vi "Animal_Deterrent_System.vi"() -> ()   [LabVIEW 2020]
uses:
  <vilib>/sound2/lvsound2.llb/Sound Output Task ID.ctl
  <vilib>/DAQmx/write.llb/DAQmx Write (Analog DBL 1Chan 1Samp).vi
  <vilib>/DAQmx/create/channels.llb/DAQmx Create Channel (AO-Voltage-Basic).vi
  <vilib>/DAQmx/miscellaneous.llb/DAQmx Fill In Error Info.vi
panel:
  out "output variable 2":dbl
  out "output variable 3":dbl
  in  "Boolean 2":bool
  in  "Boolean":bool
  out "element":path
  out "task ID":T1 format="%.0x"
  out "Avg":dbl
  in  "stop":bool
  out ".not. x?":bool
  out ".not. x? 2":bool
  out ".not. x? 4":bool
  out ".not. x? 3":bool
  out ".not. x? 6":bool
  out ".not. x? 5":bool
  out "x .and. y?":bool
  out "Light Output":dbl
  in  "physical channels 3":tag
  out "Piezo V":dbl format="%0.2f"
  out "Output variable":dbl
  out "PIR":dynamicdata(graph)
  out "Varying Peak":dbl
  out "Holding Peak":dbl
  out "IR_A":dbl
  out "IR_B":dbl
  in  "IR_A 4":bool
  in  "IR_B 5":bool
  out "Elephant 2":i32
  out "PeaFowl 2":u32
  out "Pig  2":u32
  out "Numeric 3":dbl
  in  "stop 2":bool
  out "True":bool
  out "False3":bool
  out "Pig1":bool
  out "Pig 2":bool
  out "Fowl 1":bool
  out "Fowl 2":bool
  out "Elephant 1":bool
  out "Eleplant 2":bool
  in  "Boolean 10":bool
  in  "Boolean 9":bool
  in  "Boolean 8":bool
  in  "Numeric 2":dbl
  in  "Boolean 7":bool
  out "Boolean 6":bool=TRUE
  in  "stop 3":bool
  # "ANIMAL DETERRENT SYSTEM"
  # "COUNT OF ANIMALS"
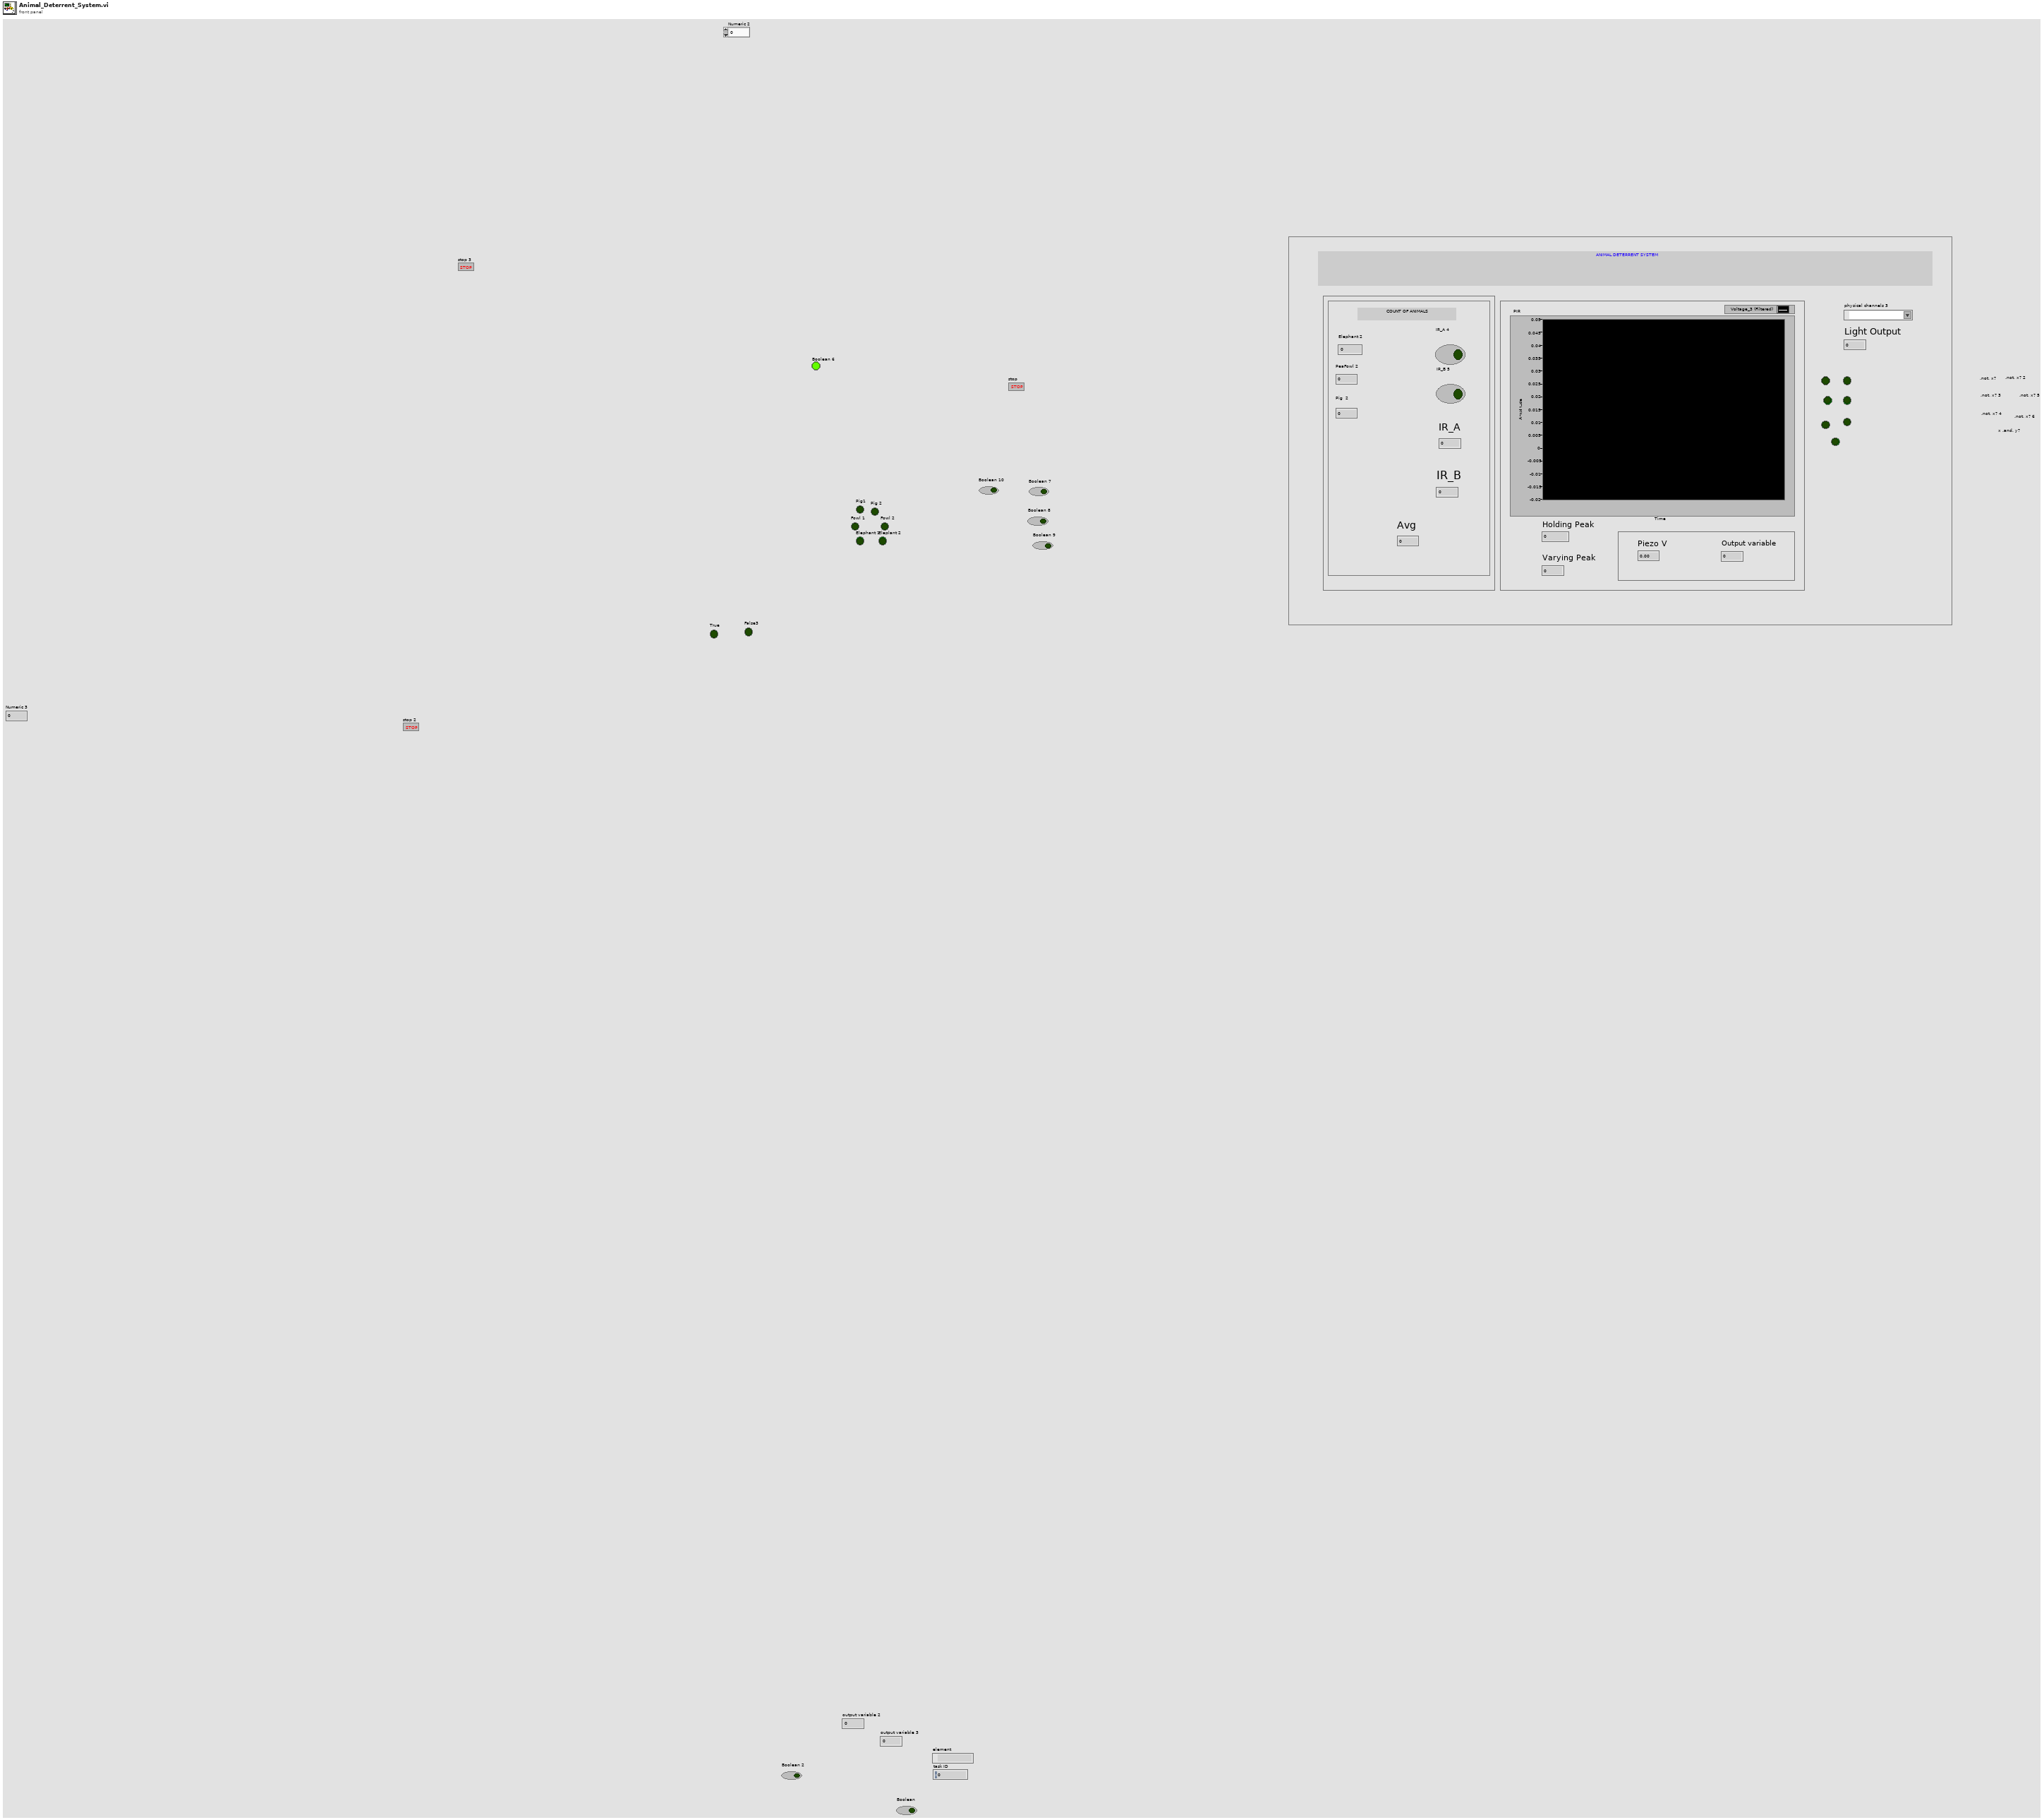
[diagram p1: front panel]
types:
  T1 = typedef "Sound Output Task ID.ctl" = u32
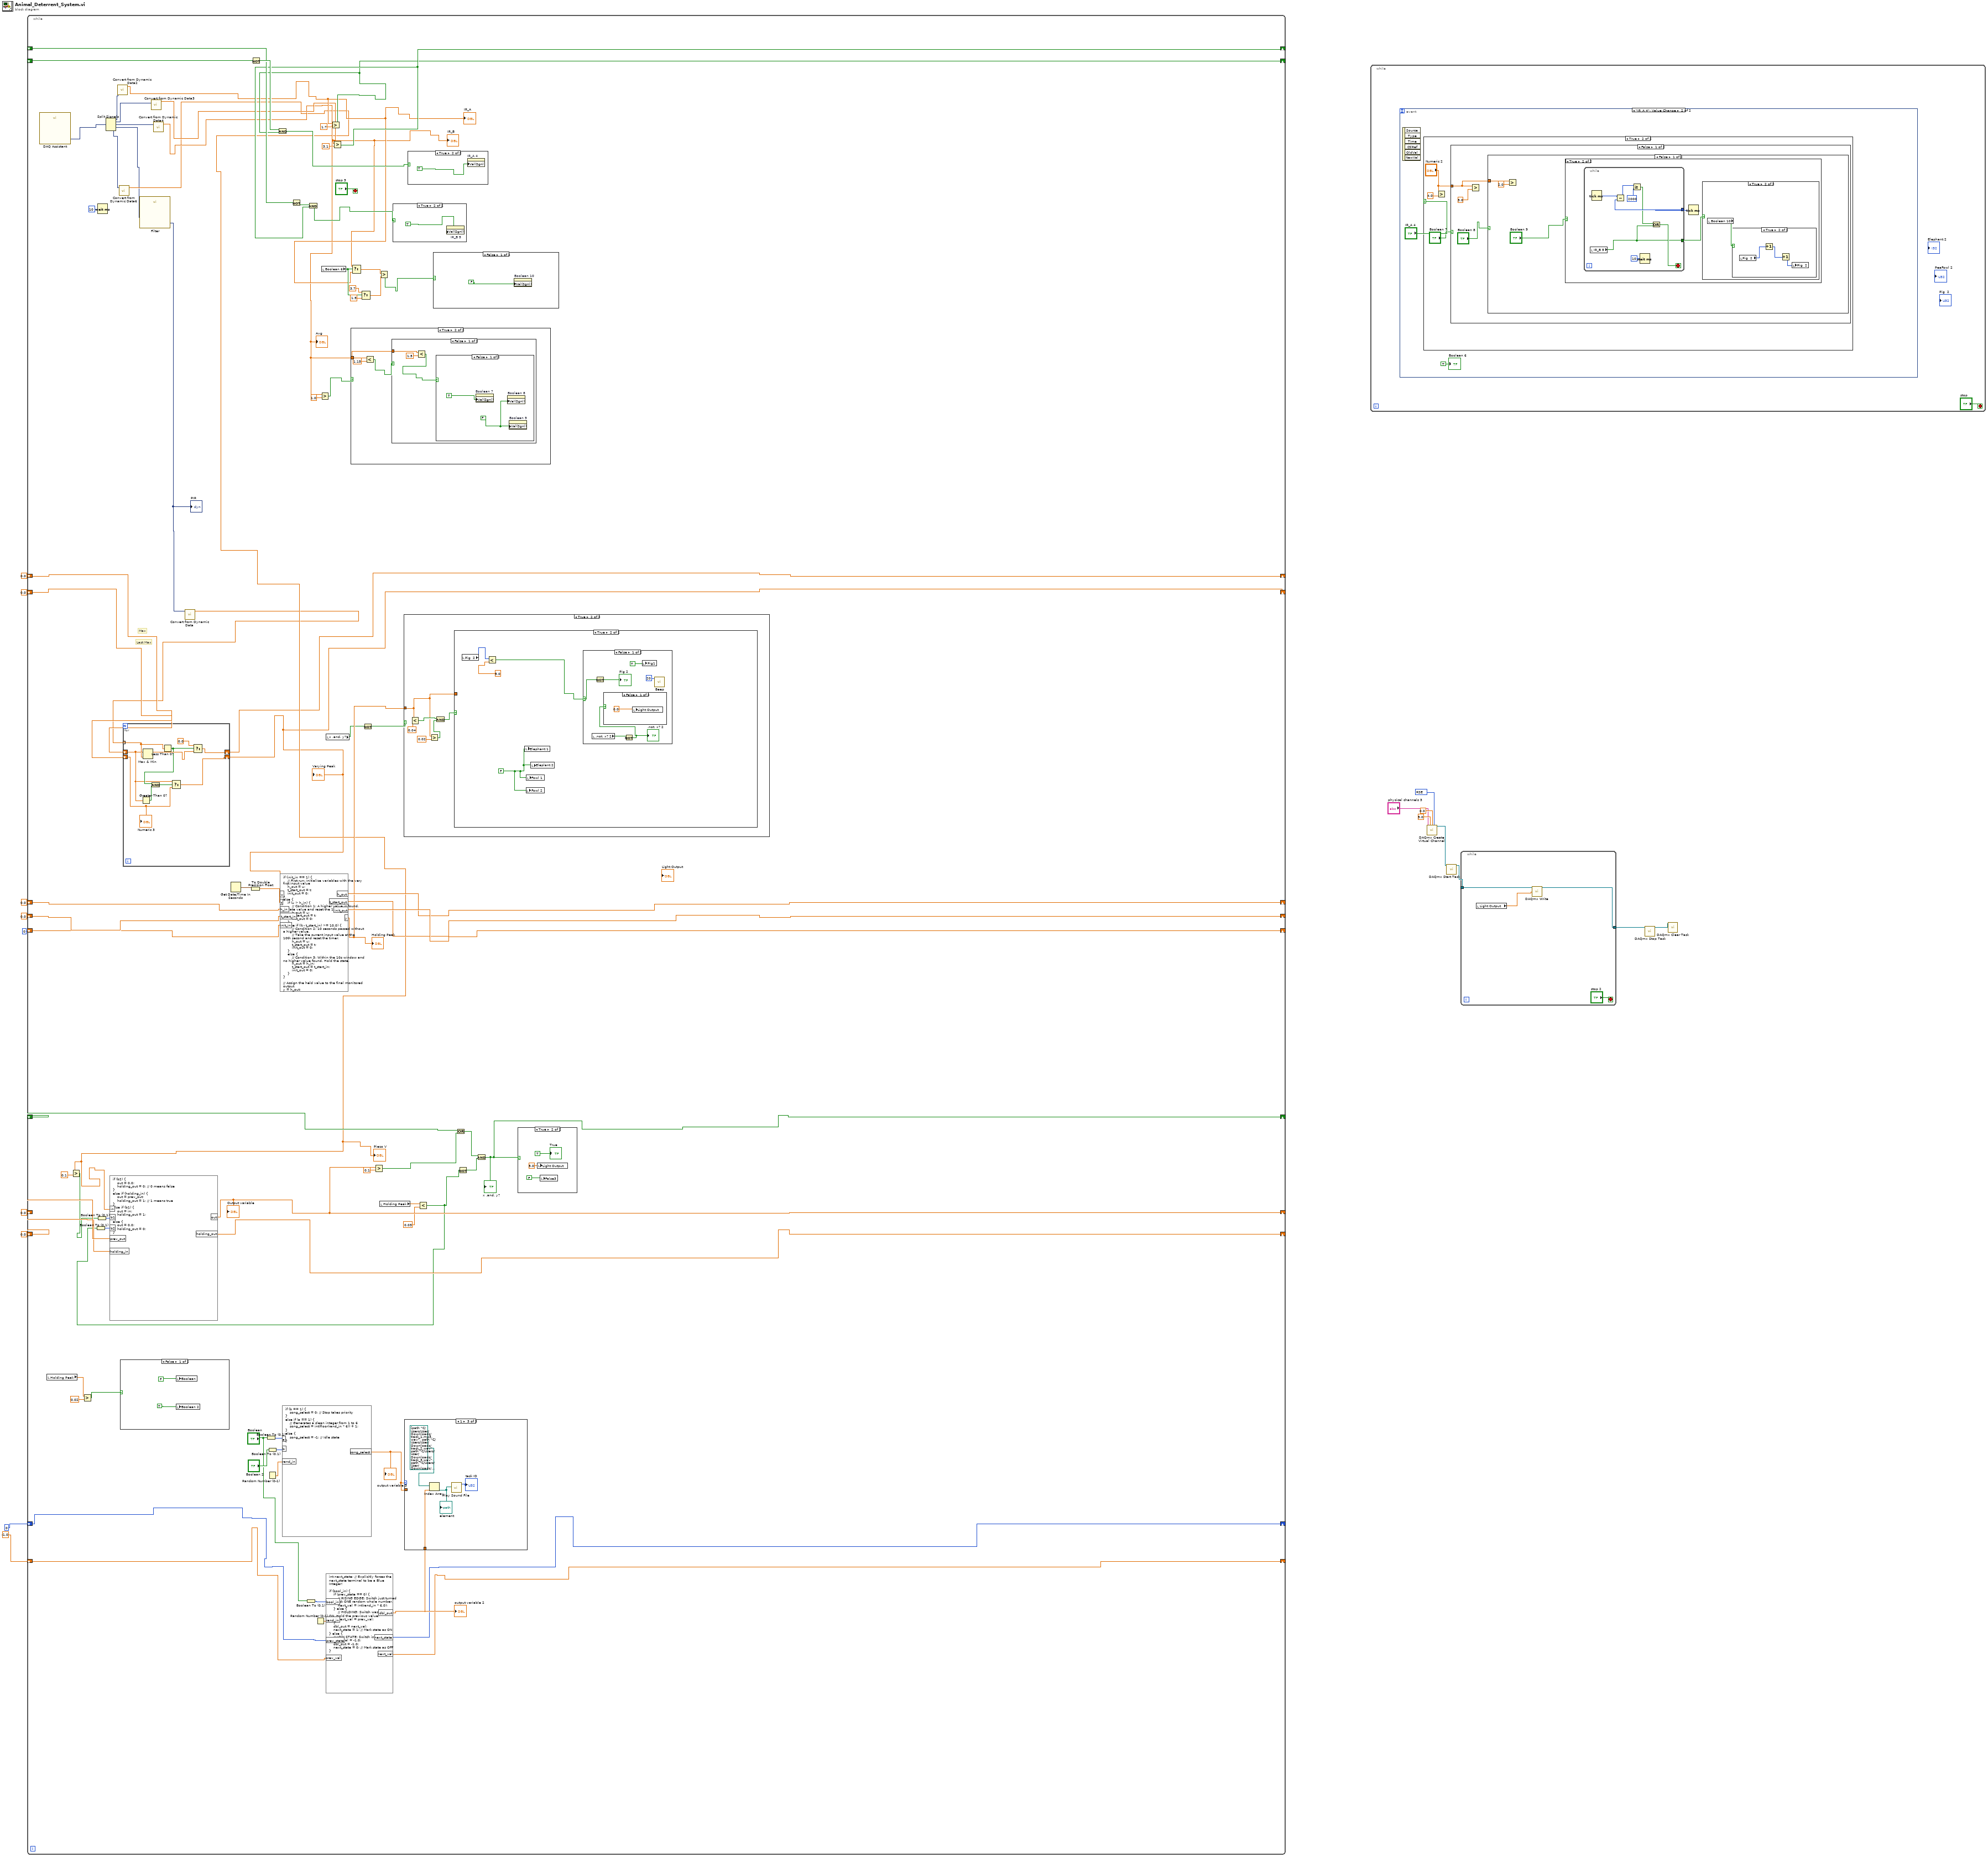
[diagram p0: block diagram]
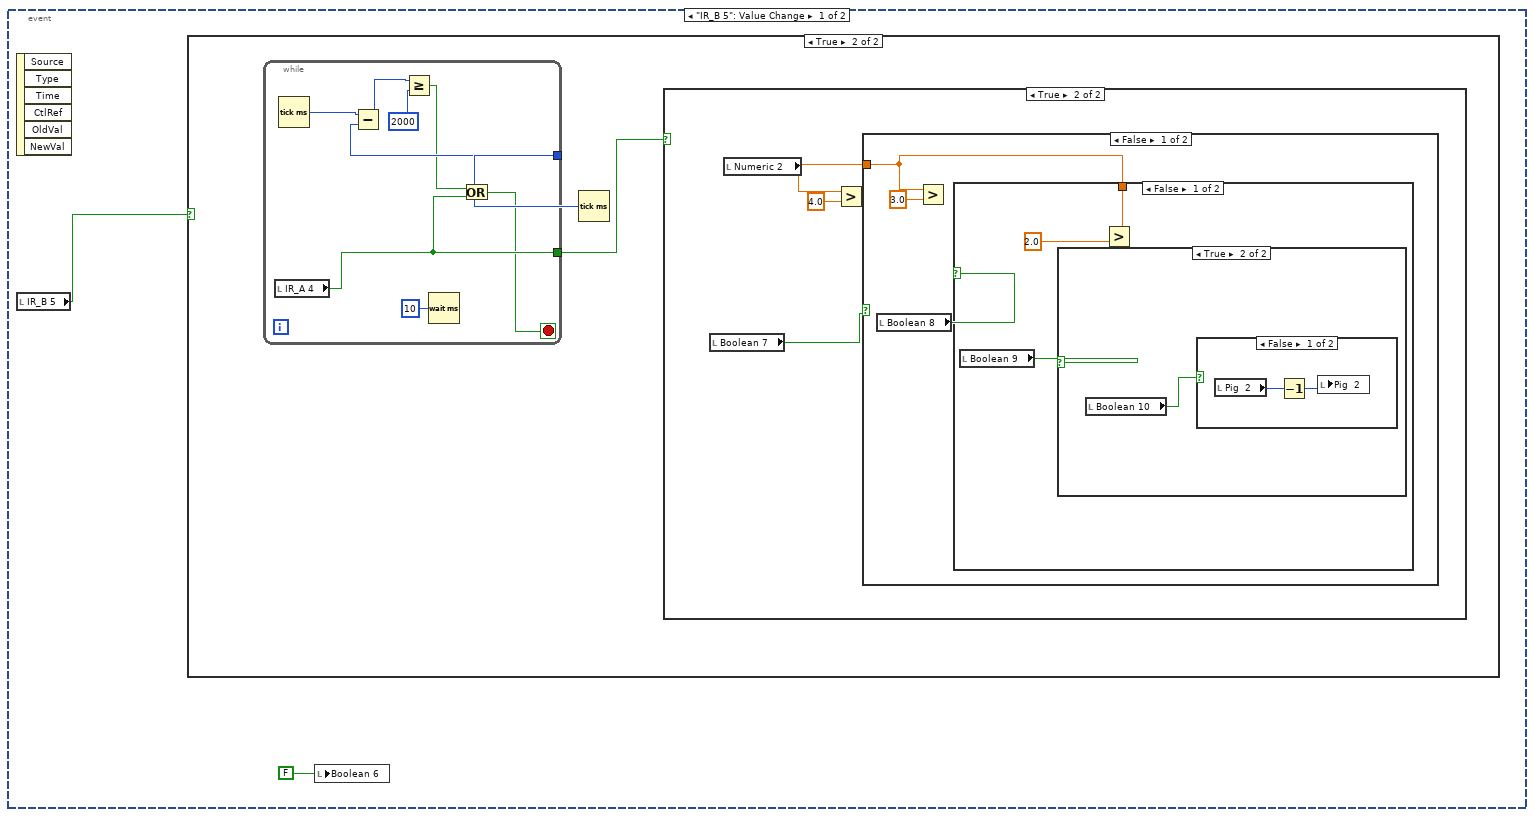
[diagram p2: hidden frame]
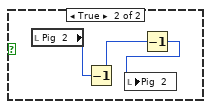
[diagram p6: hidden frame]
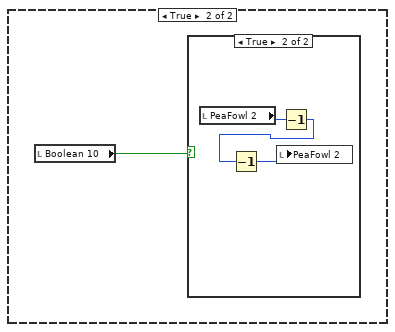
[diagram p7: hidden frame]
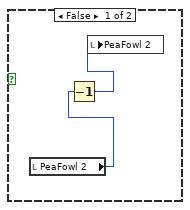
[diagram p8: hidden frame]
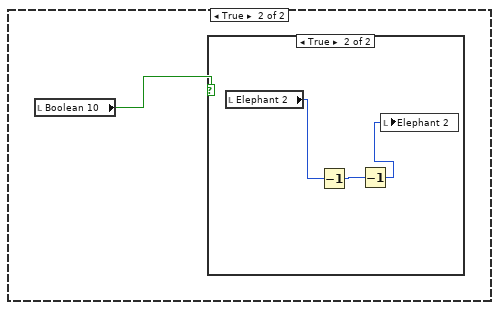
[diagram p9: hidden frame]
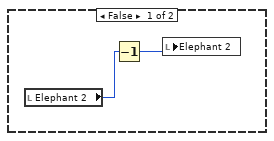
[diagram p10: hidden frame]
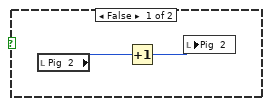
[diagram p14: hidden frame]
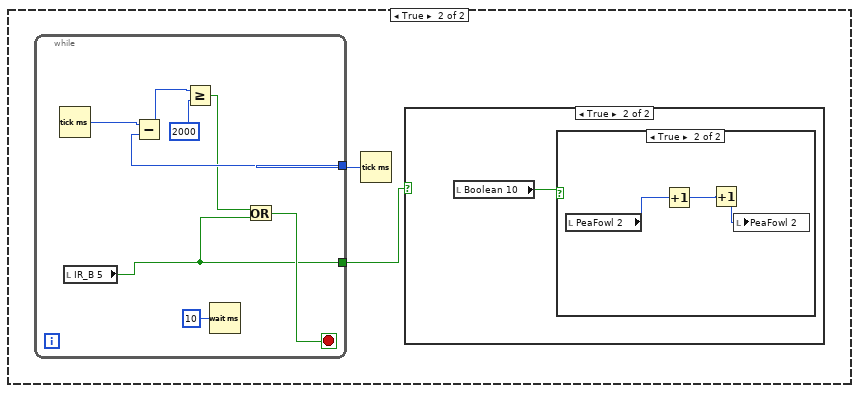
[diagram p15: hidden frame]
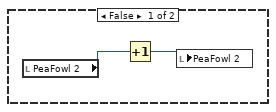
[diagram p17: hidden frame]
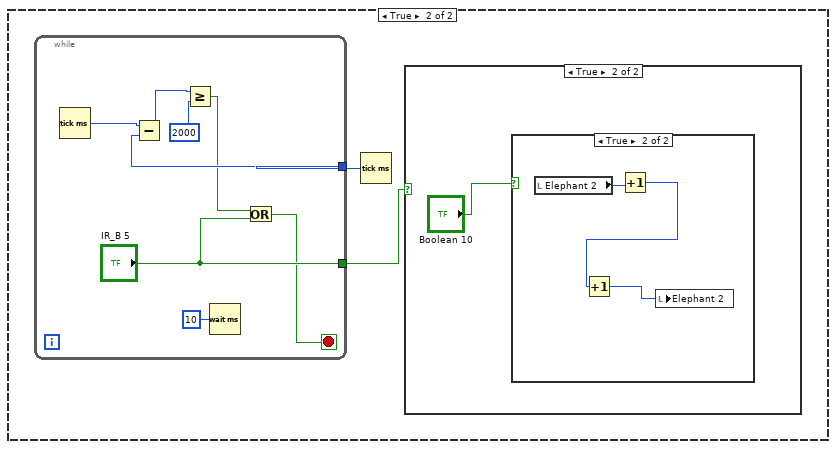
[diagram p18: hidden frame]
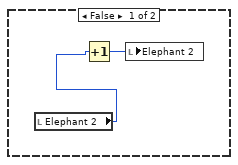
[diagram p20: hidden frame]
diagram:
  w6 = 10083 items=["Default"=-1, "RSE"=10083, "Differential"=10106, "Pseudodifferential"=12529] ("output terminal configuration")
  n1 = while {
    shift-right: [w55] -> _
    shift-left: _ -> [w94]
    shift-right: [w89] -> _
    shift-left: _ -> [w91]
    shift-right: [w41] -> _
    shift-left: 0.0 ("t") -> [w38]
    shift-right: [w40] -> _
    shift-left: 0.0 ("t") -> [w39]
    shift-right: [w71] -> _
    shift-left: 0.0 ("h_out") -> [w82]
    shift-right: [w72] -> _
    shift-left: 0.0 ("t_start_out") -> [w81]
    shift-right: [w73] -> _
    shift-left: 0 -> [w80]
    shift-right: [w74] -> _
    shift-left: _ -> [w79]
    shift-right: [w75] -> _
    shift-left: 0.0 ("out") -> [w78]
    shift-right: [w76] -> _
    shift-left: 0.0 ("holding_out") -> [w77]
    shift-right: [w22] -> _
    shift-left: 0 -> [w24]
    shift-right: [w21] -> _
    shift-left: -1.0 -> [w23]
    stop <- "stop 3" stop-if-true
    # "Last Max"
    # "Max"
    n2 = call "DAQ Assistant"() -> ("data"=w34:dynamicdata)  [unwired: 16 in, 3 out]
    n3 = local read "Holding Peak"() -> (w19:dbl)
    n4 = Greater?(x=w19, y=0.02) -> (0:w18:bool)
    n5 = Wait (ms)(milliseconds to wait=u32 10) -> ()  [unwired: 1 out]
    n6 = Split Signals(w34) -> (w47:dynamicdata, w50:dynamicdata, w49:dynamicdata, w42:dynamicdata, w48:dynamicdata)  [unwired: 5 in]
    n7 = call "Convert from Dynamic Data2"("Dynamic Data Type"=w47) -> ("Scalar"=w46:dbl)  [unwired: 3 in]
    "IR_A" <- w46
    n8 = call "Convert from Dynamic Data6"("Dynamic Data Type"=w48) -> ("Scalar"=w43:dbl)  [unwired: 3 in]
    "Piezo V" <- w43
    n9 = Greater?(x=w43, y=0.1) -> (0:w51:bool)
    n10 = Boolean To (0,1)(Boolean=w51) -> (0, 1=w62:i16)
    n11 = case shown="False" w18 {
      frame False {
        n12 = local write "Boolean"(FALSE) -> ()
        n13 = local write "Boolean 2"(TRUE) -> ()
      }
      frame True {
        n14 = local write "Boolean"(TRUE) -> ()
        n15 = local write "Boolean 2"(FALSE) -> ()
      }
    }
    n16 = call "Filter"("Signal"=w42) -> ("Filtered Signal"=w35:dynamicdata)  [unwired: 9 in, 1 out]
    "PIR" <- w35
    n17 = call "Convert from Dynamic Data3"("Dynamic Data Type"=w50) -> ("Scalar"=w45:dbl)  [unwired: 3 in]
    "IR_B" <- w45
    n18 = call "Convert from Dynamic Data4"("Dynamic Data Type"=w49) -> ("Scalar"=w44:dbl)  [unwired: 3 in]
    "Avg" <- w44
    n19 = call "Convert from Dynamic Data"("Dynamic Data Type"=w35) -> ("Array"=w36:dbl[])  [unwired: 3 in]
    n20 = for {
      shift-right: [w113] -> w41
      shift-left: w38 -> [w109]
      shift-right: [w107] -> w40
      shift-left: w39 -> [w108]
      tunnel: w36 -> [w115] mode=indexing
      n21 = Greater Than 0?(x=w109) -> (x > 0?=w112:bool)
      n22 = Max & Min(x=w115, y=w109) -> (max(x,y)=w116:dbl)  [unwired: 1 out]
      n23 = Less Than 0?(x=w115) -> (x < 0?=w111:bool)
      n24 = And(x=w111, y=w112) -> (x .and. y?=w110:bool)
      n25 = Select(t=w109, s=w110, f=w108) -> (s? t:f=w107:dbl)
      n26 = Select(t=0.0, s=w111, f=w116) -> (s? t:f=w113:dbl)
      "Numeric 3" <- w108
    }
    "Varying Peak" <- w40
    n27 = Get Date/Time In Seconds() -> (seconds since 1Jan1904=w70:timestamp)
    n28 = To Double Precision Float(number=w70) -> (double precision float=w69:dbl)
    n29 = Not(x=w94) -> (.not. x?=w93:bool)
    n30 = Boolean To (0,1)(Boolean="Boolean") -> (0, 1=w32:i16)
    n31 = Boolean To (0,1)(Boolean="Boolean 2") -> (0, 1=w31:i16)
    n32 = Random Number (0-1)() -> (number: 0 to 1=w29:dbl)
    n33 = formula code="if (init_in == 1) {\n    // First run: Initialize variables with the very first input value\n    h_out = u;\n    t_start_out = t;\n    init_out = 0;\n} \nelse {\n    if (u > h_in) {\n        // Condition 1: A higher value is found. Update value and reset the 10s timer.\n        h_out = u;\n        t_start_out = t;\n        init_out = 0;\n    } \n    else if ((t - t_start_in) >= 10.0) {\n        // Condition 2: 10 seconds passed without a higher value. \n        // Take the current input value at the 10th second and reset the timer.\n        h_out = u;\n        t_start_out = t;\n        init_out = 0;\n    } \n    else {\n        // Condition 3: Within the 10s window and no higher value found. Hold the state.\n        h_out = h_in;\n        t_start_out = t_start_in;\n        init_out = 0;\n    }\n}\n\n// Assign the held value to the final monitored output\ny = h_out;"("u"=w40, "t"=w69, "h_in"=w82, "t_start_in"=w81, "init_in"=w80) -> ("h_out"=w71:dbl, "t_start_out"=w72:dbl, "init_out"=w73:dbl, "y"=w68:dbl)
    "Holding Peak" <- w68
    n34 = formula code="if (b == 1) {\n    song_select = 0; // Stop takes priority\n} \nelse if (a == 1) {\n    // Generates a clean integer from 1 to 6\n    song_select = int(floor(rand_in * 6)) + 1; \n} \nelse {\n    song_select = -1; // Idle state\n}"("a"=w32, "b"=w31, "rand_in"=w29) -> ("song_select"=w33:dbl)
    "output variable 3" <- w33
    n35 = Not(x=w91) -> (.not. x?=w90:bool)
    n36 = Boolean To (0,1)(Boolean="Boolean") -> (0, 1=w28:i16)
    n37 = Random Number (0-1)() -> (number: 0 to 1=w27:dbl)
    n38 = Greater?(x=w44, y=1.0) -> (0:w52:bool)
    n39 = local read "Boolean 6"() -> (w83:bool)
    n40 = local read "x .and. y?"() -> (w56:bool)
    n41 = formula code="int next_state; // Explicitly forces the next_state terminal to be a Blue Integer!\n\nif (bool_in) {\n    if (prev_state == 0) {\n        // RISING EDGE: Switch just turned ON. Pick ONE random whole number.\n        next_val = int(rand_in * 6.0);\n    } else {\n        // HOLDING: Switch was already ON. Hold the previous value.\n        next_val = prev_val;\n    }\n    dbl_out = next_val;\n    next_state = 1; // Mark state as ON\n} else {\n    // LOW STATE: Switch is OFF.\n    next_val = -1.0;\n    dbl_out = -1.0;\n    next_state = 0; // Mark state as OFF\n}"("bool_in"=w28, "rand_in"=w27, "prev_state"=w24, "prev_val"=w23) -> ("dbl_out"=w26:dbl, "next_state"=w22:i32, "next_val"=w21:dbl)
    "output variable 2" <- w26
    n42 = Greater?(x=w46, y=1.7) -> (0:w55:bool)
    n43 = And(x=w93, y=w55) -> (x .and. y?=w92:bool)
    n44 = Greater?(x=w45, y=3.1) -> (0:w89:bool)
    n45 = And(x=w90, y=w89) -> (x .and. y?=w54:bool)
    n46 = case shown="True" w52 {
      tunnel: w44 -> [_ w200]
      frame False {
      }
      frame True {
        n47 = Less?(x=w200, y=1.15) -> (x < y?=w199:bool)
        n48 = case shown="False" w199 {
          tunnel: w200 -> [w203 _]
          frame False {
            n49 = Less?(x=w203, y=1.5) -> (x < y?=w202:bool)
            n50 = case shown="False" w202 {
              frame False {
                w205 = FALSE
                n51 = property on="Boolean 7" class="Bool (strict)"("Val(Sgnl)"=TRUE) -> ()  [unwired: 2 in, 2 out]
                n52 = property on="Boolean 8" class="Bool (strict)"("Val(Sgnl)"=w205) -> ()  [unwired: 2 in, 2 out]
                n53 = property on="Boolean 9" class="Bool (strict)"("Val(Sgnl)"=w205) -> ()  [unwired: 2 in, 2 out]
              }
              frame True {
                w207 = FALSE
                n54 = property on="Boolean 8" class="Bool (strict)"("Val(Sgnl)"=TRUE ("Value (Signaling)")) -> ()  [unwired: 2 in, 2 out]
                n55 = property on="Boolean 9" class="Bool (strict)"("Val(Sgnl)"=w207) -> ()  [unwired: 2 in, 2 out]
                n56 = property on="Boolean 7" class="Bool (strict)"("Val(Sgnl)"=w207) -> ()  [unwired: 2 in, 2 out]
              }
            }
          }
          frame True {
            w209 = FALSE
            n57 = property on="Boolean 9" class="Bool (strict)"("Val(Sgnl)"=TRUE) -> ()  [unwired: 2 in, 2 out]
            n58 = property on="Boolean 7" class="Bool (strict)"("Val(Sgnl)"=w209) -> ()  [unwired: 2 in, 2 out]
            n59 = property on="Boolean 8" class="Bool (strict)"("Val(Sgnl)"=w209) -> ()  [unwired: 2 in, 2 out]
          }
        }
      }
    }
    n60 = Select(t=w45, s=w83, f=w46) -> (s? t:f=w87:dbl)
    n61 = Select(t=3.7 ("y"), s=w83, f=1.9) -> (s? t:f=w84:dbl)
    n62 = Not(x=w56) -> (.not. x?=w57:bool)
    n63 = Greater?(x=w87, y=w84) -> (0:w53:bool)
    n64 = local read "Holding Peak"() -> (w64:dbl)
    n65 = case shown="True" w54 {
      frame False {
        n66 = property on="IR_B 5" class="Bool (strict)"("Val(Sgnl)"=FALSE) -> ()  [unwired: 2 in, 2 out]
      }
      frame True {
        n67 = property on="IR_B 5" class="Bool (strict)"("Val(Sgnl)"=TRUE) -> ()  [unwired: 2 in, 2 out]
      }
    }
    n68 = case shown="True" w57 {
      tunnel: w68 -> [_ w117]
      frame False {
      }
      frame True {
        n69 = Less?(x=w117, y=0.04) -> (x < y?=w120:bool)
        n70 = Greater?(x=w117, y=0.02) -> (0:w119:bool)
        n71 = And(x=w120, y=w119) -> (x .and. y?=w118:bool)
        n72 = case shown="True" w118 {
          tunnel: w117 -> [w126 _]
          frame False {
            n73 = Less?(x=w126, y=0.1) -> (x < y?=w124:bool)
            n74 = Greater?(x=w126, y=0.04) -> (0:w127:bool)
            n75 = And(x=w127, y=w124) -> (x .and. y?=w123:bool)
            n76 = case shown="True" w123 {
              tunnel: w126 -> [w130 _]
              frame False {
                n77 = Greater?(x=w130, y=0.1) -> (0:w129:bool)
                n78 = case shown="True" w129 {
                  frame False {
                    n79 = local write "Light Output"(0.0) -> ()
                  }
                  frame True {
                    w134 = TRUE
                    w135 = TRUE
                    n80 = local read "Elephant 2"() -> (w133:i32)
                    n81 = local write "Fowl 1"(w134) -> ()
                    n82 = Less?(x=w133, y=5.0) -> (x < y?=w136:bool)
                    n83 = local write "Fowl 2"(w134) -> ()
                    n84 = case shown="True" w136 {
                      selector: w136 -> [w143 w150]
                      frame False {
                        n85 = local read ".not. x? 5"() -> (w140:bool)
                        n86 = Not(x=w140) -> (.not. x?=w139:bool)
                        ".not. x? 5" <- w139
                        n87 = call <vilib>:"Beep.vi"("frequency (Hz)"=u32 60) -> ()  [unwired: 11 in]
                        n88 = case shown="True" w139 {
                          frame False {
                            n89 = local write "Light Output"(0.0 ("Light Output")) -> ()
                          }
                          frame True {
                            n90 = local write "Light Output"(3.75) -> ()
                          }
                        }
                        n91 = Not(x=w143) -> (.not. x?=→"Eleplant 2":bool)
                        n92 = local write "Elephant 1"(TRUE) -> ()
                      }
                      frame True {
                        n93 = local read ".not. x? 6"() -> (w148:bool)
                        n94 = Not(x=w148) -> (.not. x?=w147:bool)
                        ".not. x? 6" <- w147
                        n95 = case shown="True" w147 {
                          frame False {
                            n96 = local write "Light Output"(0.0 ("Light Output")) -> ()
                          }
                          frame True {
                            n97 = local write "Light Output"(3.6) -> ()
                          }
                        }
                        n98 = call <vilib>:"Beep.vi"("frequency (Hz)"=u32 50) -> ()  [unwired: 11 in]
                        n99 = local write "Eleplant 2"(FALSE) -> ()
                        "Elephant 1" <- w150
                      }
                    }
                    n100 = local write "Pig 2"(w135) -> ()
                    n101 = local write "Pig1"(w135) -> ()
                  }
                }
              }
              frame True {
                w154 = FALSE
                w155 = TRUE
                n102 = local read "PeaFowl 2"() -> (w153:u32)
                n103 = local write "Eleplant 2"(w154) -> ()
                n104 = local write "Elephant 1"(w154) -> ()
                n105 = Less?(x=w153, y=5.0) -> (x < y?=w156:bool)
                n106 = case shown="True" w156 {
                  selector: w156 -> [w163 w170]
                  frame False {
                    n107 = call <vilib>:"Beep.vi"("frequency (Hz)"=u32 40) -> ()  [unwired: 11 in]
                    n108 = local read ".not. x? 3"() -> (w160:bool)
                    n109 = Not(x=w163) -> (.not. x?=→"Fowl 2":bool)
                    n110 = Not(x=w160) -> (.not. x?=w159:bool)
                    ".not. x? 3" <- w159
                    n111 = case shown="True" w159 {
                      frame False {
                        n112 = local write "Light Output"(0.0 ("Light Output")) -> ()
                      }
                      frame True {
                        n113 = local write "Light Output"(3.45 ("Light Output")) -> ()
                      }
                    }
                    n114 = local write "Fowl 1"(TRUE) -> ()
                  }
                  frame True {
                    n115 = local read ".not. x? 4"() -> (w168:bool)
                    n116 = call <vilib>:"Beep.vi"("frequency (Hz)"=u32 30) -> ()  [unwired: 11 in]
                    n117 = Not(x=w168) -> (.not. x?=w167:bool)
                    ".not. x? 4" <- w167
                    n118 = case shown="True" w167 {
                      frame False {
                        n119 = local write "Light Output"(0.0 ("Light Output")) -> ()
                      }
                      frame True {
                        n120 = local write "Light Output"(3.3 ("Light Output")) -> ()
                      }
                    }
                    n121 = local write "Fowl 2"(FALSE) -> ()
                    "Fowl 1" <- w170
                  }
                }
                n122 = local write "Pig 2"(w155) -> ()
                n123 = local write "Pig1"(w155) -> ()
              }
            }
          }
          frame True {
            w174 = FALSE
            n124 = local read "Pig  2"() -> (w173:u32)
            n125 = Less?(x=w173, y=5.0) -> (x < y?=w175:bool)
            n126 = local write "Elephant 1"(w174) -> ()
            n127 = local write "Fowl 2"(w174) -> ()
            n128 = local write "Fowl 1"(w174) -> ()
            n129 = local write "Eleplant 2"(w174) -> ()
            n130 = case shown="False" w175 {
              selector: w175 -> [w182 w189]
              frame False {
                n131 = local read ".not. x? 2"() -> (w180:bool)
                n132 = Not(x=w182) -> (.not. x?=→"Pig 2":bool)
                n133 = Not(x=w180) -> (.not. x?=w179:bool)
                ".not. x? 2" <- w179
                n134 = case shown="False" w179 {
                  frame False {
                    n135 = local write "Light Output"(0.0) -> ()
                  }
                  frame True {
                    n136 = local write "Light Output"(1.8) -> ()
                  }
                }
                n137 = local write "Pig1"(TRUE) -> ()
                n138 = call <vilib>:"Beep.vi"("frequency (Hz)"=u32 20) -> ()  [unwired: 11 in]
              }
              frame True {
                n139 = local read ".not. x?"() -> (w187:bool)
                n140 = Not(x=w187) -> (.not. x?=w186:bool)
                ".not. x?" <- w186
                n141 = case shown="True" w186 {
                  frame False {
                    n142 = local write "Light Output"(0.0 ("Light Output")) -> ()
                  }
                  frame True {
                    n143 = local write "Light Output"(1.6) -> ()
                  }
                }
                n144 = local write "Pig 2"(FALSE) -> ()
                n145 = call <vilib>:"Beep.vi"("frequency (Hz)"=u32 10) -> ()  [unwired: 11 in]
                "Pig1" <- w189
              }
            }
          }
        }
      }
    }
    n146 = case shown="1" w33 {
      tunnel: w33 -> [_ _ _]
      tunnel: w26 -> [_ _ w105]
      frame 0 {
        n147 = local read "task ID"() -> (w102:T1)
        n148 = call <vilib>:"Sound Output Stop.vi"("task ID"=w102) -> ()  [unwired: 9 in, 2 out]
      }
      frame Default {
      }
      frame 1 {
        n149 = Index Array(array=path[] [path "C:/Users/User/Downloads/track_1.mp3.wav", path "C:/Users/User/Downloads/track_2.wav", path "C:/Users/User/Downloads/track_3.wav", path "C:/Users/User/Downloads/track_4.wav", path "C:/Users/User/Downloads/track_2.wav", path "C:/Users/User/Downloads/track_4.wav", path "C:/Users/User/Downloads/track_3.wav"], index=w105) -> (element=w104:path)
        "element" <- w104
        n150 = call <vilib>:"Play Sound File.vi"("path"=w104) -> ("task ID"=→"task ID":T1)  [unwired: 9 in, 1 out]
      }
    }
    n151 = case shown="True" w92 {
      frame False {
        n152 = property on="IR_A 4" class="Bool (strict)"("Val(Sgnl)"=FALSE) -> ()  [unwired: 2 in, 2 out]
      }
      frame True {
        n153 = property on="IR_A 4" class="Bool (strict)"("Val(Sgnl)"=TRUE) -> ()  [unwired: 2 in, 2 out]
      }
    }
    n154 = Less?(x=w64, y=0.03) -> (x < y?=w60:bool)
    n155 = Boolean To (0,1)(Boolean=w60) -> (0, 1=w61:i16)
    n156 = formula code="if (b2) {\n    out = 0.0;\n    holding_out = 0; // 0 means false\n} \nelse if (holding_in) {\n    out = prev_out;\n    holding_out = 1; // 1 means true\n} \nelse if (b1) {\n    out = in;\n    holding_out = 1; \n} \nelse {\n    out = 0.0;\n    holding_out = 0;\n}"("in"=w43, "b1"=w62, "b2"=w61, "prev_out"=w78, "holding_in"=w77) -> ("out"=w75:dbl, "holding_out"=w76:dbl)
    "Output variable" <- w75
    n157 = Greater?(x=w75, y=0.1) -> (0:w58:bool)
    n158 = case shown="False" w53 {
      frame False {
        n159 = property on="Boolean 10" class="Bool (strict)"("Val(Sgnl)"=FALSE) -> ()  [unwired: 2 in, 2 out]
      }
      frame True {
        n160 = property on="Boolean 10" class="Bool (strict)"("Val(Sgnl)"=TRUE) -> ()  [unwired: 2 in, 2 out]
      }
    }
    n161 = Or(x=w79, y=w58) -> (x .or. y?=w67:bool)
    n162 = Not(x=w60) -> (.not. x?=w66:bool)
    n163 = And(x=w67, y=w66) -> (x .and. y?=w74:bool)
    "x .and. y?" <- w74
    n164 = case shown="True" w74 {
      frame False {
        n165 = local write "True"(FALSE) -> ()
        "False3" <- TRUE
      }
      frame True {
        n166 = local write "Light Output"(5.0 ("Light Output")) -> ()
        n167 = local write "False3"(FALSE) -> ()
        "True" <- TRUE
      }
    }
  }
  n168 = while {
    stop <- "stop" stop-if-true
    n169 = event shown="[1] \"IR_A 4\": Value Change" {
      selector: _ -> [_ _]
      dyn-events: _ -> [_ _]
      timeout: _ -> [_ _]
      event "IR_B 5": Value Change {
        n170 = event-data() -> ()  [unwired: 1 in, 6 out]
        n171 = local read "IR_B 5"() -> (w217:bool)
        n172 = case shown="True" w217 {
          frame False {
          }
          frame True {
            n173 = Tick Count (ms)() -> (millisecond timer value=w219:u32)
            n174 = while {
              tunnel: w219 -> [w253]
              tunnel: [w248] -> w218
              stop <- w247 stop-if-true
              n175 = local read "IR_A 4"() -> (w248:bool)
              n176 = Tick Count (ms)() -> (millisecond timer value=w254:u32)
              n177 = Subtract(x=w254, y=w253) -> (x-y=w252:u32)
              n178 = Greater Or Equal?(x=w252, y=u32 2000) -> (x >= y?=w249:bool)
              n179 = Wait (ms)(milliseconds to wait=u32 10) -> ()  [unwired: 1 out]
              n180 = Or(x=w249, y=w248) -> (x .or. y?=w247:bool)
            }
            n181 = case shown="True" w218 {
              frame False {
              }
              frame True {
                n182 = local read "Boolean 7"() -> (w220:bool)
                n183 = local read "Numeric 2"() -> (w221:dbl)
                n184 = Greater?(x=w221, y=4.0) -> ()  [unwired: 1 out]
                n185 = case shown="False" w220 {
                  tunnel: w221 -> [w224 _]
                  frame False {
                    n186 = local read "Boolean 8"() -> (w223:bool)
                    n187 = Greater?(x=w224, y=3.0) -> ()  [unwired: 1 out]
                    n188 = case shown="False" w223 {
                      tunnel: w224 -> [w227 _]
                      frame False {
                        n189 = local read "Boolean 9"() -> (w226:bool)
                        n190 = case shown="True" w226 {
                          frame False {
                          }
                          frame True {
                            n191 = local read "Boolean 10"() -> (w229:bool)
                            n192 = case shown="False" w229 {
                              frame False {
                                n193 = local read "Pig  2"() -> (w231:u32)
                                n194 = Decrement(x=w231) -> (x-1=w230:u32)
                                n195 = local write "Pig  2"(w230) -> ()
                              }
                              frame True {
                                n196 = local read "Pig  2"() -> (w234:u32)
                                n197 = Decrement(x=w234) -> (x-1=w233:u32)
                                n198 = Decrement(x=w233) -> (x-1=w232:u32)
                                n199 = local write "Pig  2"(w232) -> ()
                              }
                            }
                          }
                        }
                        n200 = Greater?(x=w227, y=2.0) -> ()  [unwired: 1 out]
                      }
                      frame True {
                        n201 = local read "Boolean 10"() -> (w235:bool)
                        n202 = case shown="True" w235 {
                          frame False {
                            n203 = local read "PeaFowl 2"() -> (w237:u32)
                            n204 = Decrement(x=w237) -> (x-1=w236:u32)
                            n205 = local write "PeaFowl 2"(w236) -> ()
                          }
                          frame True {
                            n206 = local read "PeaFowl 2"() -> (w240:u32)
                            n207 = Decrement(x=w240) -> (x-1=w239:u32)
                            n208 = Decrement(x=w239) -> (x-1=w238:u32)
                            n209 = local write "PeaFowl 2"(w238) -> ()
                          }
                        }
                      }
                    }
                  }
                  frame True {
                    n210 = local read "Boolean 10"() -> (w241:bool)
                    n211 = case shown="True" w241 {
                      frame False {
                        n212 = local read "Elephant 2"() -> (w242:i32)
                        n213 = Decrement(x=w242) -> (x-1=w243:i32)
                        n214 = local write "Elephant 2"(w243) -> ()
                      }
                      frame True {
                        n215 = local read "Elephant 2"() -> (w246:i32)
                        n216 = Decrement(x=w246) -> (x-1=w245:i32)
                        n217 = Decrement(x=w245) -> (x-1=w244:i32)
                        n218 = local write "Elephant 2"(w244) -> ()
                      }
                    }
                  }
                }
              }
            }
          }
        }
        n219 = local write "Boolean 6"(FALSE) -> ()
      }
      event "IR_A 4": Value Change {
        n220 = event-data() -> ()  [unwired: 1 in, 6 out]
        n221 = case shown="True" "IR_A 4" {
          frame False {
          }
          frame True {
            n222 = Greater?(x="Numeric 2", y=4.0) -> ()  [unwired: 1 out]
            n223 = case shown="False" "Boolean 7" {
              tunnel: "Numeric 2" -> [w261 _]
              frame False {
                n224 = Greater?(x=w261, y=3.0) -> ()  [unwired: 1 out]
                n225 = case shown="False" "Boolean 8" {
                  tunnel: w261 -> [w265 _]
                  frame False {
                    n226 = Greater?(x=w265, y=2.0) -> ()  [unwired: 1 out]
                    n227 = case shown="True" "Boolean 9" {
                      frame False {
                      }
                      frame True {
                        n228 = Tick Count (ms)() -> (millisecond timer value=w267:u32)
                        n229 = while {
                          tunnel: w267 -> [w280]
                          tunnel: [w274] -> w266
                          stop <- w275 stop-if-true
                          n230 = local read "IR_B 5"() -> (w274:bool)
                          n231 = Tick Count (ms)() -> (millisecond timer value=w281:u32)
                          n232 = Subtract(x=w281, y=w280) -> (x-y=w279:u32)
                          n233 = Greater Or Equal?(x=w279, y=u32 2000) -> (x >= y?=w276:bool)
                          n234 = Wait (ms)(milliseconds to wait=u32 10) -> ()  [unwired: 1 out]
                          n235 = Or(x=w276, y=w274) -> (x .or. y?=w275:bool)
                        }
                        n236 = case shown="True" w266 {
                          frame False {
                          }
                          frame True {
                            n237 = local read "Boolean 10"() -> (w268:bool)
                            n238 = case shown="True" w268 {
                              frame False {
                                n239 = local read "Pig  2"() -> (w269:u32)
                                n240 = Increment(x=w269) -> (x+1=w270:u32)
                                n241 = local write "Pig  2"(w270) -> ()
                              }
                              frame True {
                                n242 = local read "Pig  2"() -> (w272:u32)
                                n243 = Increment(x=w272) -> (x+1=w271:u32)
                                n244 = Increment(x=w271) -> (x+1=w273:u32)
                                n245 = local write "Pig  2"(w273) -> ()
                              }
                            }
                          }
                        }
                      }
                    }
                  }
                  frame True {
                    n246 = Tick Count (ms)() -> (millisecond timer value=w283:u32)
                    n247 = while {
                      tunnel: w283 -> [w296]
                      tunnel: [w290] -> w282
                      stop <- w291 stop-if-true
                      n248 = Tick Count (ms)() -> (millisecond timer value=w297:u32)
                      n249 = local read "IR_B 5"() -> (w290:bool)
                      n250 = Subtract(x=w297, y=w296) -> (x-y=w295:u32)
                      n251 = Greater Or Equal?(x=w295, y=u32 2000) -> (x >= y?=w292:bool)
                      n252 = Wait (ms)(milliseconds to wait=u32 10) -> ()  [unwired: 1 out]
                      n253 = Or(x=w292, y=w290) -> (x .or. y?=w291:bool)
                    }
                    n254 = case shown="True" w282 {
                      frame False {
                      }
                      frame True {
                        n255 = local read "Boolean 10"() -> (w284:bool)
                        n256 = case shown="True" w284 {
                          frame False {
                            n257 = local read "PeaFowl 2"() -> (w285:u32)
                            n258 = Increment(x=w285) -> (x+1=w286:u32)
                            n259 = local write "PeaFowl 2"(w286) -> ()
                          }
                          frame True {
                            n260 = local read "PeaFowl 2"() -> (w287:u32)
                            n261 = Increment(x=w287) -> (x+1=w288:u32)
                            n262 = Increment(x=w288) -> (x+1=w289:u32)
                            n263 = local write "PeaFowl 2"(w289) -> ()
                          }
                        }
                      }
                    }
                  }
                }
              }
              frame True {
                n264 = Tick Count (ms)() -> (millisecond timer value=w299:u32)
                n265 = while {
                  tunnel: w299 -> [w312]
                  tunnel: ["IR_B 5"] -> w298
                  stop <- w306 stop-if-true
                  n266 = Tick Count (ms)() -> (millisecond timer value=w313:u32)
                  n267 = Subtract(x=w313, y=w312) -> (x-y=w311:u32)
                  n268 = Greater Or Equal?(x=w311, y=u32 2000) -> (x >= y?=w308:bool)
                  n269 = Wait (ms)(milliseconds to wait=u32 10) -> ()  [unwired: 1 out]
                  n270 = Or(x=w308, y="IR_B 5") -> (x .or. y?=w306:bool)
                }
                n271 = case shown="True" w298 {
                  frame False {
                  }
                  frame True {
                    n272 = case shown="True" "Boolean 10" {
                      frame False {
                        n273 = local read "Elephant 2"() -> (w301:i32)
                        n274 = Increment(x=w301) -> (x+1=w302:i32)
                        n275 = local write "Elephant 2"(w302) -> ()
                      }
                      frame True {
                        n276 = local read "Elephant 2"() -> (w305:i32)
                        n277 = Increment(x=w305) -> (x+1=w304:i32)
                        n278 = Increment(x=w304) -> (x+1=w303:i32)
                        n279 = local write "Elephant 2"(w303) -> ()
                      }
                    }
                  }
                }
              }
            }
          }
        }
        "Boolean 6" <- TRUE
      }
    }
  }
  n280 = call-poly <vilib>:"DAQmx Create Virtual Channel.vi"("maximum value"=5.0, "minimum value"=0.0, "output terminal configuration"=w6, "physical channels"="physical channels 3") -> ("task out"=w10:refnum<k21>)  [unwired: 10 in, 1 out]
  n281 = call <vilib>:"DAQmx Start Task.vi"("task/channels in"=w10) -> ("task out"=w9:refnum<k21>)  [unwired: 13 in, 1 out]
  n282 = while {
    tunnel: w9 -> [w316]
    tunnel: [w315] -> w8
    stop <- "stop 2" stop-if-true
    n283 = local read "Light Output"() -> (w314:dbl)
    n284 = call-poly <vilib>:"DAQmx Write.vi"("task/channels in"=w316, "data"=w314) -> ("task out"=w315:refnum<k21>)  [unwired: 11 in, 2 out]
  }
  n285 = call <vilib>:"DAQmx Stop Task.vi"("task/channels in"=w8) -> ("task out"=w7:refnum<k21>)  [unwired: 13 in, 1 out]
  n286 = call <vilib>:"DAQmx Clear Task.vi"("task in"=w7) -> ()  [unwired: 14 in, 1 out]
